vi "Delete Last Item.vi"(8 "error in (no error)":errorcluster, 10 "Removed VI":refnum<class "Standard VI Type.lvclass">, 11 "Data Cluster":T1) -> (0 "error out":errorcluster, 3 "Module Data":T1)   [LabVIEW 2020, in "Peek Window.lvlib"]
uses:
  Peek Window.lvlib
  MHL Data Cluster.ctl
  VI Types/Standard VI Type/Standard VI Type.lvclass
  VI Types/Standard VI Type/Standard VI Type.lvclass/Standard VI Type.ctl
  VI Types/Standard VI Type/Read Full Qualified Name.vi
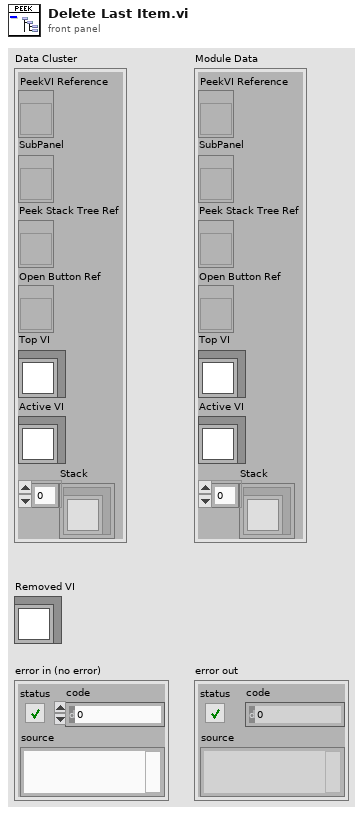
[diagram p1: front panel]
types:
  T1 = typedef "Peek Window.lvlib/MHL Data Cluster.ctl" = cluster{"PeekVI Reference":refnum<vi>, "SubPanel":refnum<vi>, "Peek Stack Tree Ref":refnum<vi>, "Open Button Ref":refnum<vi>, "Top VI":refnum<class "Standard VI Type.lvclass">, "Active VI":refnum<class "Standard VI Type.lvclass">, "Stack":refnum<class "Standard VI Type.lvclass">[]}
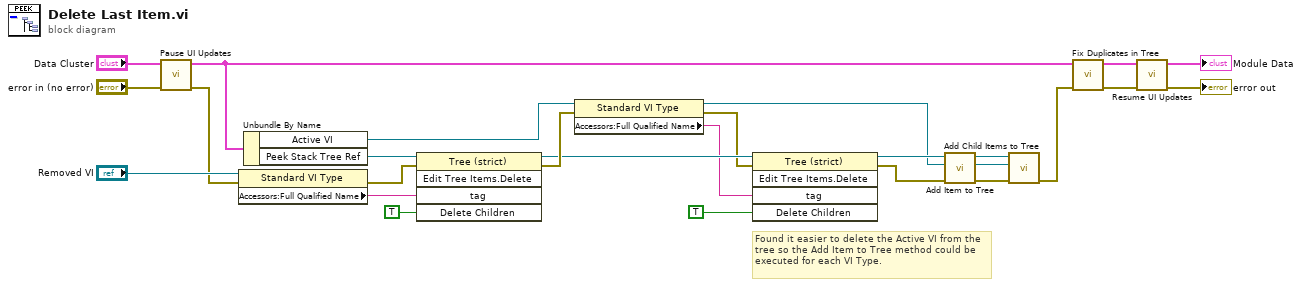
[diagram p0: block diagram]
diagram:
  # "Found it easier to delete the Active VI from the tree so the Add Item to Tree method could be executed for each VI Type."
  n1 = call "Pause UI Updates.vi"("error in"="error in (no error)", "Module Data"="Data Cluster") -> ("error out"=w14:errorcluster, "Module Data"=w18:T1)  [unwired: 8 in]
  n2 = property class="Standard VI Type"(reference="Removed VI", error in=w14) -> (error out=w13:errorcluster, "Accessors:Full Qualified Name"=w15:string)  [unwired: 1 out]
  n3 = Unbundle By Name(w18) -> ("Active VI"=w17:refnum<class "Standard VI Type.lvclass">, "Peek Stack Tree Ref"=w26:refnum<vi>)
  n4 = invoke class="Tree (strict)" method="Edit Tree Items.Delete"(reference=w26, error in=w13, "tag"=w15, "Delete Children"=TRUE) -> (reference out=w11:refnum<vi>, error out=w16:errorcluster)  [unwired: 1 in, 3 out]
  n5 = property class="Standard VI Type"(reference=w17, error in=w16) -> (reference out=w6:refnum<class "Standard VI Type.lvclass">, error out=w9:errorcluster, "Accessors:Full Qualified Name"=w10:string)
  n6 = invoke class="Tree (strict)" method="Edit Tree Items.Delete"(reference=w11, error in=w9, "tag"=w10, "Delete Children"=TRUE) -> (reference out=w8:refnum<vi>, error out=w4:errorcluster)  [unwired: 1 in, 3 out]
  n7 = call-dynamic "Add Item to Tree.vi"("error in (no error)"=w4, "Standard VI Type in"=w6, "Tree Ref in"=w8) -> ("error out"=w3:errorcluster, "Standard VI Type out"=w5:refnum<class "Standard VI Type.lvclass">, "Tree Ref out"=w7:refnum<vi>)  [unwired: 5 in, 1 out]
  n8 = call-dynamic "Add Child Items to Tree.vi"("error in (no error)"=w3, "Standard VI Type in"=w5, "Tree Ref in"=w7) -> ("error out"=w2:errorcluster)  [unwired: 6 in, 2 out]
  n9 = call "Fix Duplicates in Tree.vi"("error in (no error)"=w2, "Data in"=w18) -> ("error out"=w1:errorcluster, "Data out"=w19:T1)  [unwired: 8 in]
  n10 = call "Resume UI Updates.vi"("error in"=w1, "Module Data"=w19) -> ("error out"=→"error out":errorcluster, "Module Data"=→"Module Data":T1)  [unwired: 8 in]
